vi "Configure Range Table (Spurious Emissions - Frequency And Bandwidth).vi"(0 "VISA resource name":refnum<visa-resource-name>, 1 "Enable Auto Resolution Bandwidth":bool[](array[boolean])=[TRUE, TRUE], 2 "Manual Resolution Bandwidth":i32[](array[numeric])=[1000000, 1000000], 5 "Enable Range":bool[](array[boolean])=[TRUE, TRUE], 7 "Start Frequency":i32[](array[numeric])=[1920000000, 1920000000], 9 "Stop Frequency":i32[](array[numeric])=[1980000000, 1980000000], 11 "error in (no error)":errorcluster, 12 "Enable Auto Video Bandwidth":bool[](array[boolean])=[TRUE, TRUE], 13 "Manual Video Bandwidth":i32[](array[numeric])=[1000000, 1000000]) -> (4 "VISA resource name out":refnum<visa-resource-name>, 15 "error out":errorcluster)   [LabVIEW 2014, in "Agilent ESA PSA Series.lvlib"]
doc: "Configures the frequency,resolution,bandwidth of the measurement."
uses:
  Agilent ESA PSA Series.lvlib
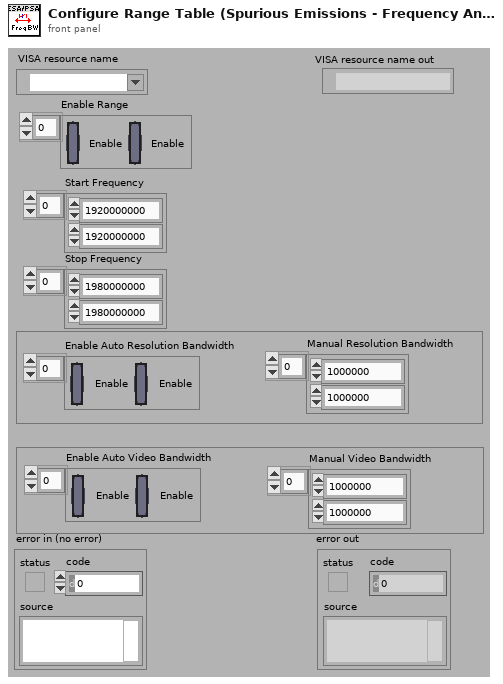
[diagram p1: front panel]
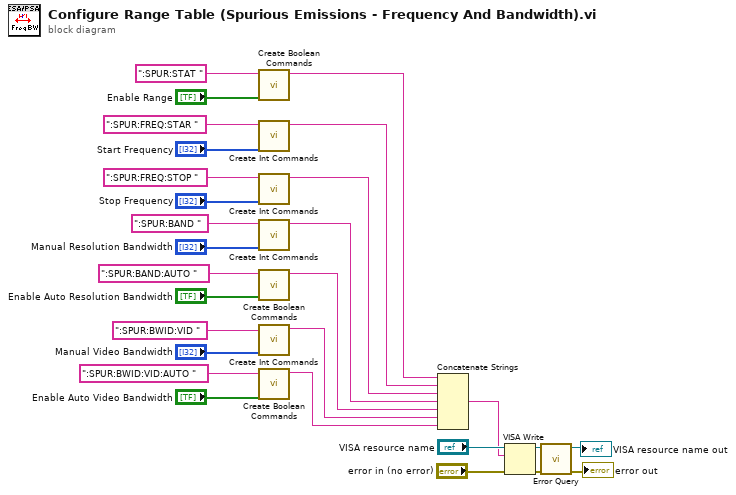
[diagram p0: block diagram]
diagram:
  n1 = call "Create Boolean Commands.vi"("States"="Enable Range", "Command"=":SPUR:STAT ") -> ("Result String"=w9:string)  [unwired: 9 in]
  n2 = call "Create Int Commands.vi"("Values"="Start Frequency", "Commands"=":SPUR:FREQ:STAR ") -> ("Result"=w8:string)  [unwired: 9 in]
  n3 = call "Create Int Commands.vi"("Values"="Stop Frequency", "Commands"=":SPUR:FREQ:STOP ") -> ("Result"=w7:string)  [unwired: 9 in]
  n4 = call "Create Int Commands.vi"("Values"="Manual Resolution Bandwidth", "Commands"=":SPUR:BAND ") -> ("Result"=w6:string)  [unwired: 9 in]
  n5 = call "Create Boolean Commands.vi"("States"="Enable Auto Resolution Bandwidth", "Command"=":SPUR:BAND:AUTO ") -> ("Result String"=w5:string)  [unwired: 9 in]
  n6 = call "Create Int Commands.vi"("Values"="Manual Video Bandwidth", "Commands"=":SPUR:BWID:VID ") -> ("Result"=w4:string)  [unwired: 9 in]
  n7 = call "Create Boolean Commands.vi"("States"="Enable Auto Video Bandwidth", "Command"=":SPUR:BWID:VID:AUTO ") -> ("Result String"=w3:string)  [unwired: 9 in]
  n8 = Concatenate Strings(w9, w8, w7, w6, w5, w4, w3) -> (w24:string)
  n9 = VISA Write(VISA resource name="VISA resource name", write buffer=w24, error in (no error)="error in (no error)") -> (VISA resource name out=w2:refnum<visa-resource-name>, error out=w1:errorcluster)  [unwired: 1 out]
  n10 = call "Error Query.vi"("error in (no error)"=w1, "VISA resource name"=w2) -> ("error out"=→"error out":errorcluster, "VISA resource name out"=→"VISA resource name out":refnum<visa-resource-name>)  [unwired: 6 in, 2 out]
